vi "API_DB.GetLocationStatusFromDB.vi"(0 "Database in":refnum<class "Database.lvclass">, 1 "Wait (F)":bool, 2 "InventoryRecord.Location.Module":u16, 5 "Table":string, 7 "InventoryRecord.Stocker":T1 items=["Main", "Exp1", "Exp2"], 11 "error in (no error)":errorcluster, 12 "Timeout (ms)":u32, 13 "InventoryRecord.Location.Row":u16, 14 "InventoryRecord.Location.Column":u16) -> (4 "Database out":refnum<class "Database.lvclass">, 6 "Slot":string, 15 "error out":errorcluster)   [LabVIEW 2020, in "Database.lvclass"]
doc: "Developed by Kevin Thompson\nkevin@thompsonengineering.net\n\nCopyright 2018\nThompson Engineering, LLC"
uses:
  Database.lvclass
  DataTypes/Stocker--Enum.ctl
  DataTypes/AsynCmd_Temp01--enum.ctl
  DataTypes/GenericQuery--Cluster.ctl
  DataTypes/SQLQuery--Enum.ctl
  DataTypes/InventoryRecord--Cluster.ctl
  DataTypes/Module--Cluster.ctl
  DataTypes/LocationStatus--Enum.ctl
  Database.lvclass/Database.ctl
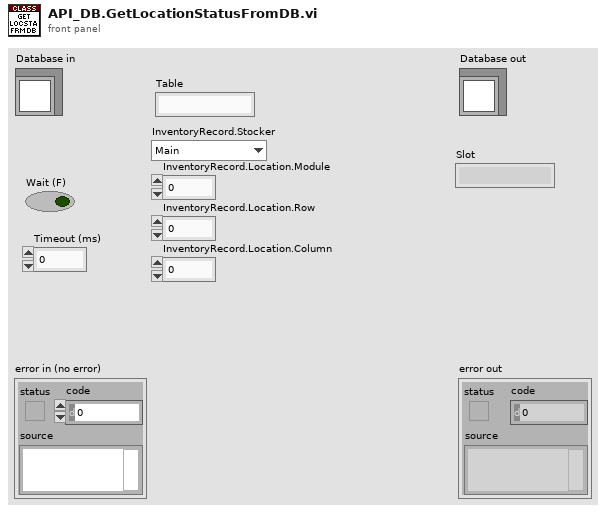
[diagram p1: front panel]
types:
  T1 = typedef "Stocker--Enum.ctl" = u16
  T2 = typedef "SQLQuery--Enum.ctl" = enum16{"GetInventoryRecordFromDB", "GetReticleInfoFromDB", "GetLocationStatusFromDB", "UpdateInventoryRecord", "UpdateLocationStatus", "UpdateReticleLocationStatus", "AddReticleInDB", "RemoveReticleAtLocation", "RemoveReticleUsingReticleID", "GetLocationForReticleID", "GetAllLocations", "GetAllEmptyLocations", "GetAllLocationsInStocker", "GetAllFullLocations", "GetAllFullLocationsInStocker", "GetAllDisabledLocations", "GetAllDisabledLocationsInStocker", "FindFirstSlot"}
  T3 = typedef "GenericQuery--Cluster.ctl" = cluster{"Query":T2, "Table":string, "InventoryRecord":T4}
  T4 = typedef "InventoryRecord--Cluster.ctl" = cluster{"ReticleID":string, "Stocker":T1, "Location":T5, "LocationStatus":T6, "EquipmentID":string, "LocationID":string}
  T5 = typedef "Module--Cluster.ctl" = cluster{"Module":u16, "Row":u16, "Column":u16}
  T6 = typedef "LocationStatus--Enum.ctl" = enum16{"Disabled/Unusable", "Full", "Empty"}
  T7 = typedef "Database.lvclass/AsynCmd_Temp01--enum.ctl" = enum16{"DB.DeleteRecord", "DB.UpdateRecord", "DB.InsertRecord", "DB.SelectRecord", "DB.ExecuteSQLCommand", "DB.FindFirstSlot", "DB.GenericSQLQuery"}
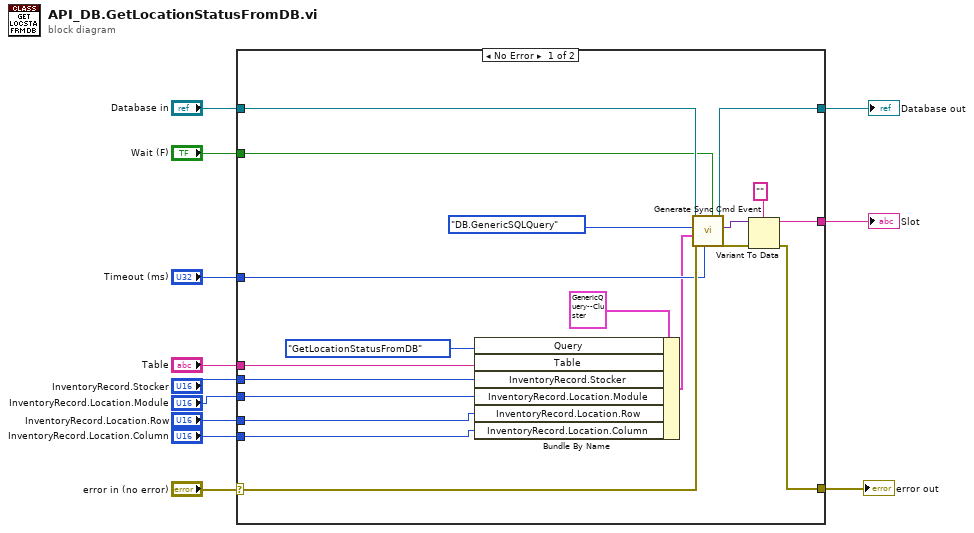
[diagram p0: block diagram]
diagram:
  n1 = case shown="No Error" "error in (no error)" {
    selector: "error in (no error)" -> [w29 w33]
    tunnel: [w24 w33] -> w11
    tunnel: [w30 w32] -> w9
    tunnel: "Database in" -> [w31 w32]
    tunnel: [w26 _] -> w6
    tunnel: "Wait (F)" -> [w23 _]
    tunnel: "Timeout (ms)" -> [w22 _]
    tunnel: "Table" -> [w17 _]
    tunnel: "InventoryRecord.Stocker" -> [w16 _]
    tunnel: "InventoryRecord.Location.Module" -> [w15 _]
    tunnel: "InventoryRecord.Location.Row" -> [w14 _]
    tunnel: "InventoryRecord.Location.Column" -> [w13 _]
    frame No Error {
      n2 = Bundle By Name(cluster=T3 {"Query"=enum."GetInventoryRecordFromDB", "Table"="", "InventoryRecord"={"ReticleID"="", "Stocker"=0, "Location"={"Module"=0, "Row"=0, "Column"=0}, "LocationStatus"=enum."Disabled/Unusable", "EquipmentID"="", "LocationID"=""}}, "Query"=SQLQuery--Enum."GetLocationStatusFromDB", "Table"=w17, "InventoryRecord.Stocker"=w16, "InventoryRecord.Location.Module"=w15, "InventoryRecord.Location.Row"=w14, "InventoryRecord.Location.Column"=w13) -> (w18:T3)
      n3 = call "Generate Sync Cmd Event.vi"("Wait (F)"=w23, "Timeout (ms)"=w22, "error in (no error)"=w29, "vData"=w18, "AsyncCmd"=AsynCmd_Temp01--enum."DB.GenericSQLQuery", "Database in"=w31) -> ("error out"=w25:errorcluster, "Return Value"=w27:variant, "Database out"=w30:refnum<class "Database.lvclass">)  [unwired: 3 in]
      n4 = Variant To Data(error in=w25, type="", Variant=w27) -> (data=w26:string, error out=w24:errorcluster)
    }
    frame Error {
    }
  }
  "error out" <- w11
  "Database out" <- w9
  "Slot" <- w6
